vi "ZeroTimeGraph.vi"() -> ()   [LabVIEW 2012]
panel:
  in  "ZeroTimeGraph":dbl
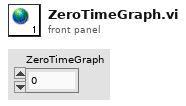
[diagram p1: front panel]
diagram:
